vi "nextSiblingNodeData.vi"(8 "error in (no error)":errorcluster caption="errorIn", 11 "siblingNode":refnum<k20>) -> (0 "error out":errorcluster caption="errorOut", 2 "data":string, 3 "childNode":refnum<k20>)   [LabVIEW 2017]
uses:
  <vilib>/xml/Close Reference(Node).vi
  <vilib>/xml/NI_XML.lvlib
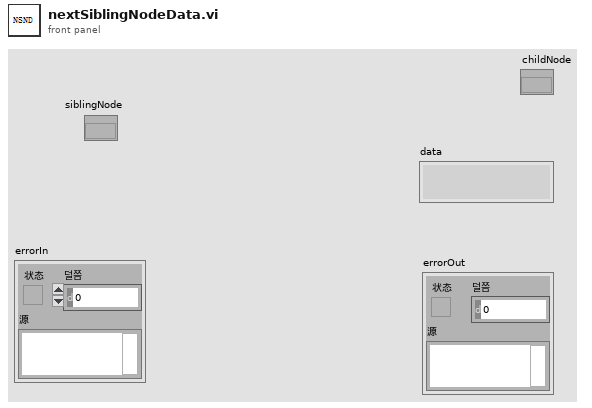
[diagram p1: front panel]
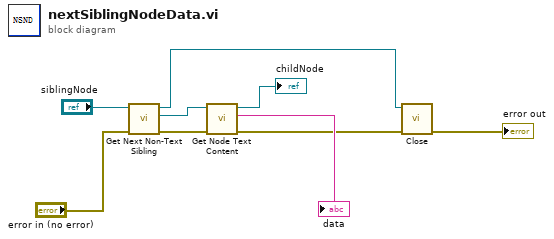
[diagram p0: block diagram]
diagram:
  n1 = call <vilib>:"Get Next Non-Text Sibling.vi"("error in (no error)"="error in (no error)", "node in"="siblingNode") -> ("error out"=w9:errorcluster, "sibling node"=w8:refnum<k20>, "node out"=w2:refnum<k20>)  [unwired: 6 in, 1 out]
  n2 = call <vilib>:"Get Node Text Content.vi"("error in (no error)"=w9, "node in"=w8) -> ("error out"=w3:errorcluster, "node text"=→"data":string, "node out"=→"childNode":refnum<k20>)  [unwired: 7 out]
  n3 = call-poly <vilib>:"Close.vi"("error in (no error)"=w3, "node"=w2) -> ("error out"=→"error out":errorcluster)  [unwired: 7 in]
